vi "Write loopTimer.vi"(10 "LoopTimer.lvclass":refnum<class "ILoopTimer.lvclass">, 11 "Model in":refnum<class "Model.lvclass">) -> (3 "Model out":refnum<class "Model.lvclass">)   [LabVIEW 2015, in "Model.lvclass"]
uses:
  Model.lvclass
  ComponentTemplateCore/ComponentModel/ComponentModelRT/LoopTimer/ILoopTimer/ILoopTimer.lvclass
  Model.lvclass/Model.ctl
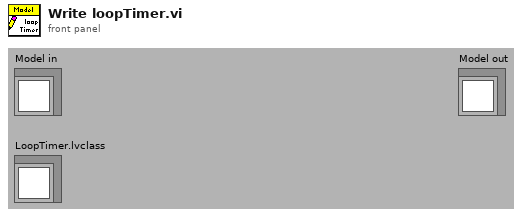
[diagram p1: front panel]
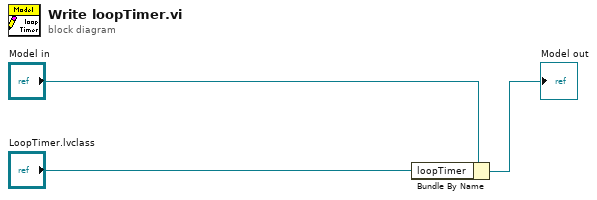
[diagram p0: block diagram]
diagram:
  n1 = Bundle By Name(cluster="Model in", "loopTimer"="LoopTimer.lvclass") -> (→"Model out":refnum<class "Model.lvclass">)
